vi "Offset Column Headers.vi"(9 "Channel Type":string, 11 "Source":string) -> (2 "Column Headers":string[][](array[string]))   [LabVIEW 2009]
panel:
  in  "Row Header\nRoot":string[](array[string])=["Offset", "Current"]
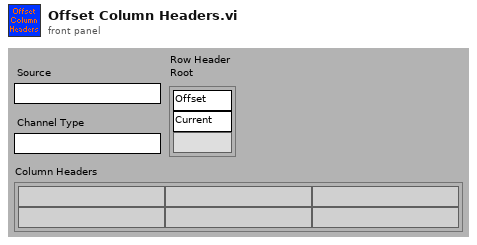
[diagram p1: front panel]
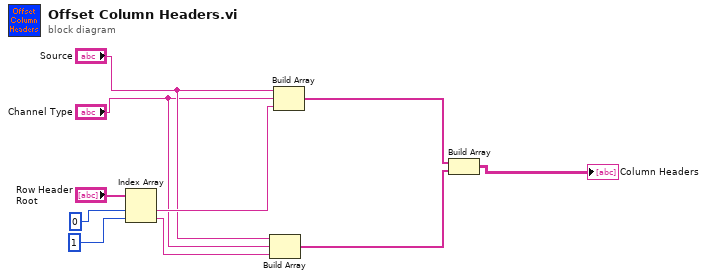
[diagram p0: block diagram]
diagram:
  n1 = Index Array(array="Row Header\nRoot", index #1=0 ("index"), index #2=1 ("index")) -> (element #1=w7:string, element #2=w6:string)
  n2 = Build Array("Source", "Channel Type", w6) -> (w2:string[])
  n3 = Build Array("Source", "Channel Type", w7) -> (w3:string[])
  n4 = Build Array(w3, w2) -> (→"Column Headers":string[][])
